vi "ORS_PathAddNumber_noExt.vi"(7 "format string":string="-%d", 10 "number":i32, 11 "path":path=path "E:/temp/test.dat") -> (3 "path output":path=path "E:/temp/2009.04.30_15.58.02_test.dat")   [LabVIEW 2021]
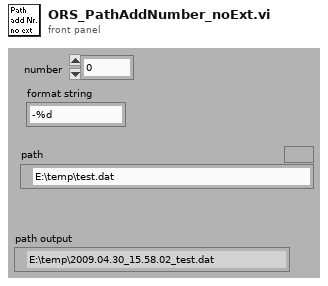
[diagram p1: front panel]
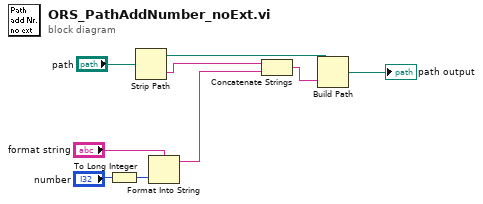
[diagram p0: block diagram]
diagram:
  n1 = To Long Integer(number="number") -> (32bit integer=w7:i32)
  n2 = Strip Path(path="path") -> (stripped path=w4:path, name=w3:string)
  n3 = Format Into String(format string="format string", w7) -> (resulting string=w2:string)  [unwired: 2 in, 1 out]
  n4 = Concatenate Strings(w3, w2) -> (w1:string)
  n5 = Build Path(base path=w4, name or relative path=w1) -> (appended path=→"path output":path)
